vi "Insert Lines.vi"(0 "Display State In":T1={"logTable"=refnum, "max items"=500, "displaydata"=[], "data"=[], "Auto Scroll"=TRUE, "current item"=500, "col headers"=[], "Add to Top"=TRUE, "Auto resize"=TRUE, "col size"=[], "filters"=[], "color cells"=[]}, 5 "Lines":string[][](array[string]), 9 "Container State":T3, 11 "error in (no error)":errorcluster) -> (4 "Display State Out":T1={"logTable"=refnum, "max items"=500, "displaydata"=[], "data"=[], "Auto Scroll"=TRUE, "current item"=500, "col headers"=[], "Add to Top"=TRUE, "Auto resize"=TRUE, "col size"=[], "filters"=[], "color cells"=[]}, 15 "error out":errorcluster)   [LabVIEW 2017, in "UI-DisplayTable(dev).xctl"]
uses:
  UI-DisplayTable(dev).xctl
  <vilib>/_xctls/Container State.ctl
  State.ctl
  Support/DEF-Filter.ctl
  <vilib>/_xctls/XControlSupport.lvlib
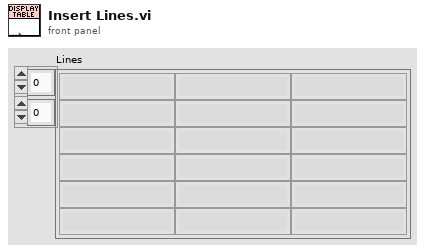
[diagram p1: front panel]
types:
  T1 = typedef "UI-DisplayTable(dev).xctl/State.ctl" = cluster{"logTable":refnum<vi>, "max items":i32, "displaydata":string[][], "data":string[][], "Auto Scroll":bool, "current item":i32, "col headers":string[], "Add to Top":bool, "Auto resize":bool, "col size":i32[], "filters":T2[], "color cells":cluster{"color cell":cluster{"Column":string, "Value":string, "Highlight Column":string}, "Color Box":u32}[]}
  T2 = typedef "UI-DisplayTable(dev).xctl/DEF-Filter.ctl" = cluster{"column":string, "value":string[]}
  T3 = typedef "XControlSupport.lvlib/Container State.ctl" = cluster{"Indicator?":bool, "Run Mode?":bool, " Refnum":refnum<vi>}
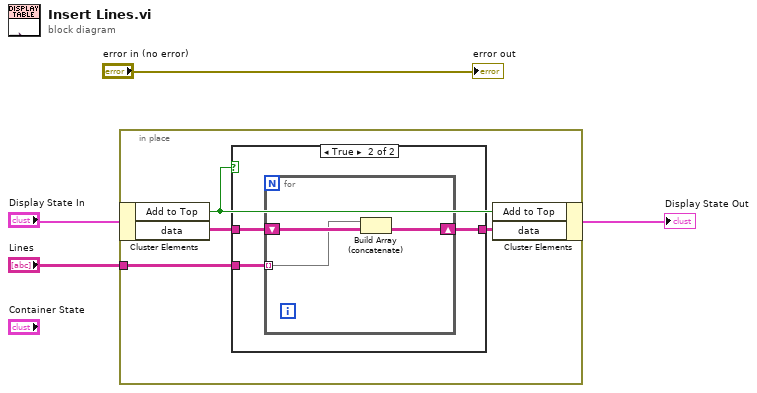
[diagram p0: block diagram]
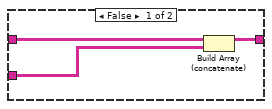
[diagram p2: hidden frame]
diagram:
  n1 = in-place {
    in-place-border: "Lines" -> [w7]
    n2 = in-place-cluster #1("Display State In") -> ("Add to Top"=w5:bool, "data"=w8:string[][])
    n3 = case shown="True" w5 {
      tunnel: w8 -> [w11 w14]
      tunnel: w7 -> [w10 w12]
      tunnel: [w9 w13] -> w6
      frame False {
        n4 = Build Array (concatenate)(w11, w10) -> (w9:string[][])
      }
      frame True {
        n5 = for {
          tunnel: w12 -> [w15] mode=indexing
          shift-right: [w16] -> w13
          shift-left: w14 -> [w17]
          n6 = Build Array (concatenate)(w15, w17) -> (w16:string[][])
        }
      }
    }
    n7 = in-place-cluster #1("Add to Top"=w5, "data"=w6) -> (→"Display State Out":T1)
  }
  "error out" <- "error in (no error)"
